vi "Get Frequency.vi"(8 "error in (no error)":errorcluster, 11 "niDTS GNSS Dut in":refnum<class "niDTS GNSS Dut.lvclass">) -> (0 "error out":errorcluster, 2 "Frequency (Hz)":dbl=1575420000.0 format="%#_6p", 3 "niDTS GNSS Dut out":refnum<class "niDTS GNSS Dut.lvclass">)   [LabVIEW 2015, in "niDTS GNSS.lvlib" / "niDTS GNSS Dut.lvclass"]
uses:
  niDTS GNSS Dut.lvclass
  niDTS GNSS Dut.lvclass/niDTS GNSS Dut.ctl
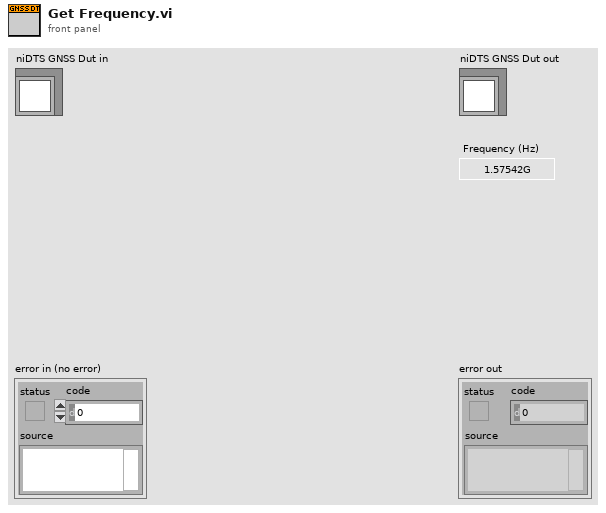
[diagram p1: front panel]
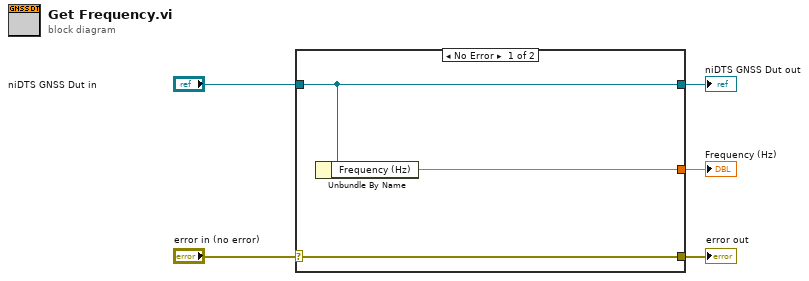
[diagram p0: block diagram]
diagram:
  n1 = case shown="No Error" "error in (no error)" {
    selector: "error in (no error)" -> [w8 w9]
    tunnel: [w8 w9] -> w4
    tunnel: [w7 w10] -> w2
    tunnel: "niDTS GNSS Dut in" -> [w7 w10]
    tunnel: [w6 _] -> w1
    frame No Error {
      n2 = Unbundle By Name(w7) -> ("Frequency (Hz)"=w6:dbl)
    }
    frame Error {
    }
  }
  "error out" <- w4
  "niDTS GNSS Dut out" <- w2
  "Frequency (Hz)" <- w1
